vi "Limited Equal Check.vi"(3 "decplaceaccurracy":u32=3 caption="Decimal Place Accuracy (3)", 4 "number2":dbl caption="Number 2", 5 "number1":dbl caption="Number 1") -> (0 "number2OUT":dbl caption="Number 2", 1 "equal?":bool caption="Equal", 2 "number1OUT":dbl caption="Number 1")   [LabVIEW 2009]
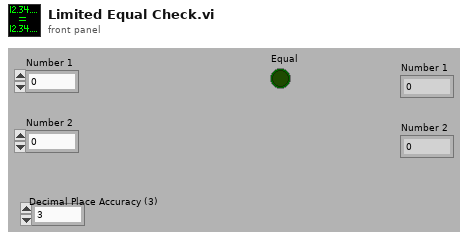
[diagram p1: front panel]
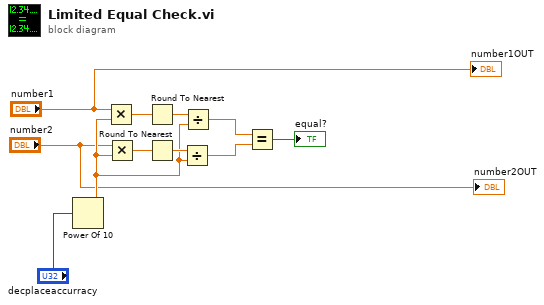
[diagram p0: block diagram]
diagram:
  n1 = Power Of 10(x="decplaceaccurracy") -> (10^x=w6:dbl)
  n2 = Multiply(x="number1", y=w6) -> (x*y=w10:dbl)
  n3 = Multiply(x="number2", y=w6) -> (x*y=w9:dbl)
  n4 = Round To Nearest(number=w10) -> (nearest integer value=w7:dbl)
  n5 = Round To Nearest(number=w9) -> (nearest integer value=w8:dbl)
  n6 = Divide(x=w8, y=w6) -> (x/y=w5:dbl)
  n7 = Divide(x=w7, y=w6) -> (x/y=w4:dbl)
  n8 = Equal?(x=w4, y=w5) -> (x = y?=→"equal?":bool)
  "number1OUT" <- "number1"
  "number2OUT" <- "number2"
